vi "Decades125.vi"(6 "NPointsPerDecade":u16(ring) items=["1", "3", "9", "20"], 9 "BaseUnit":dbl=1e-12 min=1e-12 max=0.001, 11 "NumberDecades":i32=1 min=1 max=10) -> (3 "output array":dbl[](array[numeric]) format="%#_6p")   [LabVIEW 2024]
uses:
  <vilib>/Analysis/1siggen.llb/Ramp Pattern by Samples.vi
  <vilib>/Analysis/NI_AALBase.lvlib
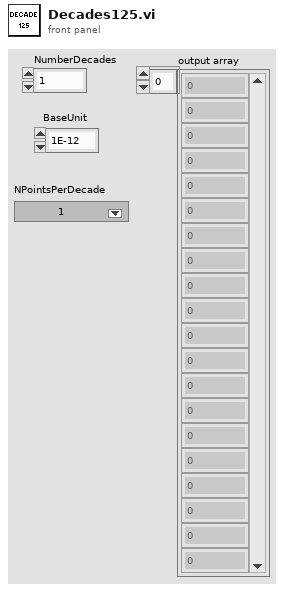
[diagram p1: front panel]
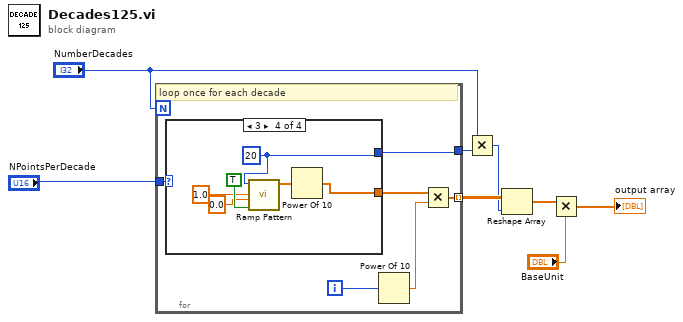
[diagram p0: block diagram]
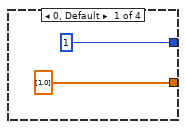
[diagram p2: hidden frame]
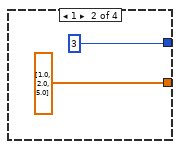
[diagram p3: hidden frame]
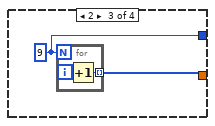
[diagram p4: hidden frame]
diagram:
  n1 = for {
    N: "NumberDecades" -> [_]
    tunnel: [w11] -> w8 mode=indexing
    tunnel: "NPointsPerDecade" -> [w10]
    tunnel: [w9] -> w1
    i -> [w14]
    # "loop once for each decade"
    n2 = case shown="3" w10 {
      tunnel: [dbl[] [1.0] dbl[] [1.0, 2.0, 5.0] w20 w24] -> w13
      tunnel: [1 3 ("y") w19 w23] -> w9
      frame 0, Default {
      }
      frame 1 {
      }
      frame 2 {
        w19 = 9
        n3 = for {
          N: w19 -> [_]
          tunnel: [w21] -> w20 mode=indexing
          i -> [w22]
          n4 = Increment(x=w22) -> (x+1=w21:i32)
        }
      }
      frame 3 {
        w23 = 20 ("samples")
        n5 = call-poly <vilib>:"Ramp Pattern.vi"("exclude end?"=TRUE, "start"=0.0, "end"=1.0, "samples"=w23) -> ("Ramp Pattern"=w28:dbl[])  [unwired: 6 in, 1 out]
        n6 = Power Of 10(x=w28) -> (10^x=w24:dbl[])
      }
    }
    n7 = Power Of 10(x=w14) -> (10^x=w12:dbl)
    n8 = Multiply(x=w13, y=w12) -> (x*y=w11:dbl[])
  }
  n9 = Multiply(x="NumberDecades", y=w1) -> (x*y=w6:i32)
  n10 = Reshape Array(w8, w6) -> (w5:dbl[])
  n11 = Multiply(x=w5, y="BaseUnit") -> (x*y=→"output array":dbl[])
